vi "Audio Test.Generate Sine Sweep, Finite Steps.vi"(8 "error in":errorcluster, 10 "Cal Data":path, 11 "Sine Sweep Params":T1={"Duration"=2.1, "Amplitude"=1.0, "FreqStart"=20000.0, "FreqEnd"=100.0, "SampleRate"=44100.0, "StepCnt"=120, "FreqSpacing"=enum."Logarithmic", "Settling"={"Time"=0.0, "Cycles"=1.0}, "Measurement"={"Time"=0.001, "Cycles"=10.0}, "SyncPulseEn"=FALSE} {"Measurement"."Cycles" min=5.0 max=1000.0 step=1.0; "Measurement"."Time" min=0.0 max=5.0 step=0.0001 format="%.3f s"; "Settling"."Cycles" min=0.0 max=100.0 step=0.5; "Settling"."Time" min=0.0 max=5.0 step=0.0001 format="%.3f s"; "StepCnt" min=1; "Amplitude" min=0.0 max=1.0 step=0.1}) -> (0 "error out":errorcluster, 1 "Total Samples":i32, 2 "Output Wvfrm":waveform(dbl)(graph), 3 "SigConfig":refnum<class "SV Discrete Sweep.lvclass">, 4 "Cal Output Wvfrm":waveform(dbl)(graph))   [LabVIEW 2018]
uses:
  TypeDefs/AudioTest.Config, Sine Sweep Params_V2.ctl
  <vilib>/addons/_NISVFA/_Generation/Signal Generation/SV Discrete Sweep/SV Discrete Sweep.lvclass
  C:/Program Files (x86)/National Instruments/LabVIEW 2018/vi.lib/addons/_NISVFA/_Generation/Signal Generation/SV Signal/SV Signal.lvclass
  C:/Program Files (x86)/National Instruments/LabVIEW 2018/vi.lib/addons/_NISVFA/_Generation/Signal Generation/SV Function/SV Function.lvclass
  <vilib>/addons/_NISVFA/_Generation/Signal Generation/SV Signal/SV Signal.lvclass/SV Signal.ctl
  <vilib>/addons/_NISVFA/_Generation/Signal Generation/SV Discrete Sweep/SV Discrete Sweep.lvclass/SV Discrete Sweep.ctl
  <vilib>/addons/_NISVFA/_Generation/Signal Generation/SV Signal/Write Leading Synchronization Pulse Enable.vi
  <vilib>/addons/_NISVFA/_Generation/Signal Generation/SV Signal/Write Synchronization Pulse Duration.vi
  <vilib>/addons/_NISVFA/_Generation/Signal Generation/SV Signal/Write Synchronization Pulse Level.vi
  <vilib>/addons/_NISVFA/_Generation/Signal Generation/SV Signal/Write Synchronization Pulse Type.vi
  <vilib>/addons/_NISVFA/_Generation/Signal Generation/SV Discrete Sweep/Read All Frequencies and Amplitudes.vi
  <vilib>/addons/_NISVFA/_Generation/Signal Generation/SV Discrete Sweep/Write All Frequencies and Amplitudes.vi
  <vilib>/addons/_NISVFA/_Generation/Signal Generation/SV Discrete Sweep/Read Frequencies and Amplitudes.vi
  <vilib>/addons/_NISVFA/_Generation/Signal Generation/SV Discrete Sweep/Configure Frequency Sweep at Constant Amplitude.vi
  <vilib>/addons/_NISVFA/_Generation/Signal Generation/SV Signal/Write Ramp Parameters.vi
  <vilib>/addons/_NISVFA/_Generation/Signal Generation/SV Signal/Write DC Offset.vi
  <vilib>/addons/_NISVFA/_Generation/Signal Generation/SV Signal/Write Measurement Duration.vi
  <vilib>/addons/_NISVFA/_Generation/Signal Generation/SV Function/Write Measurement Cycles.vi
  <vilib>/addons/_NISVFA/_Generation/Signal Generation/SV Signal/Write Pre-Measurement Settling Duration.vi
  <vilib>/addons/_NISVFA/_Generation/Signal Generation/SV Function/Write Pre-Measurement Settling Cycles.vi
  <vilib>/addons/_NISVFA/_Generation/Signal Generation/SV Signal/Write Sample Rate.vi
  <vilib>/addons/_NISVFA/_Generation/Signal Generation/SV Signal/SV Signal.lvclass
panel:
  out "size(s)":i32
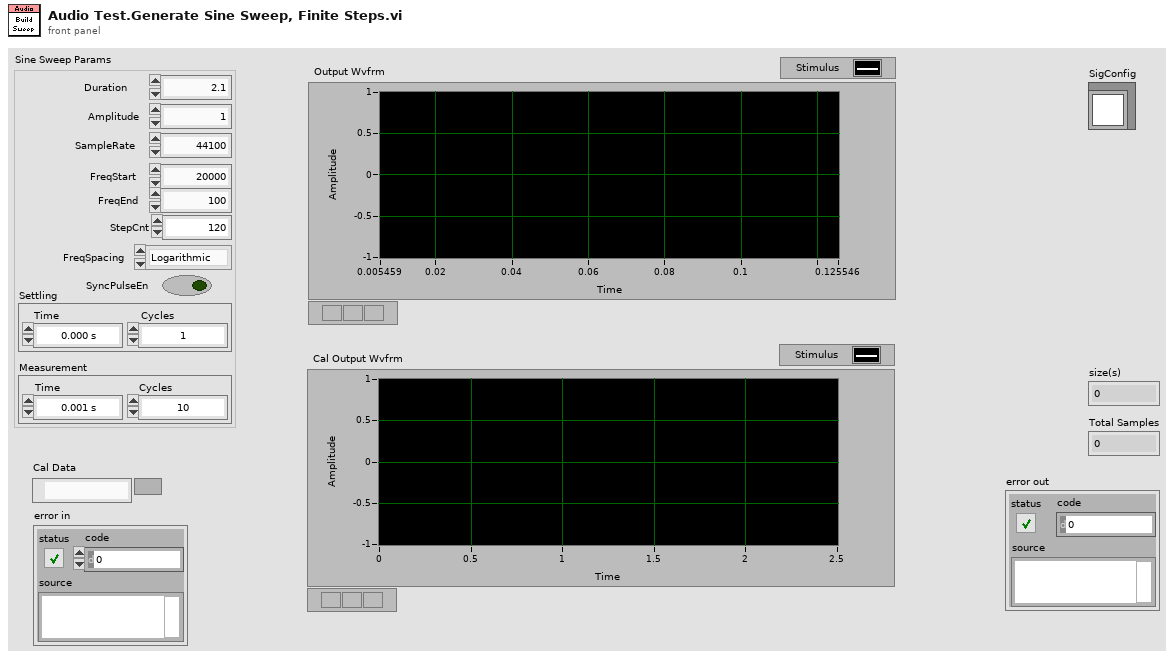
[diagram p1: front panel]
types:
  T1 = typedef "AudioTest.Config, Sine Sweep Params_V2.ctl" = cluster{"Duration":dbl, "Amplitude":dbl, "FreqStart":dbl, "FreqEnd":dbl, "SampleRate":dbl, "StepCnt":i32, "FreqSpacing":enum16{"Linear", "Logarithmic"}, "Settling":cluster{"Time":dbl, "Cycles":dbl}, "Measurement":cluster{"Time":dbl, "Cycles":dbl}, "SyncPulseEn":bool}
  T2 = enum16{"Noise", "MLS", "Chirp", "Monopulse", "Custom"}
  T3 = cluster{"profile":enum16{"Linear", "Half cosine"}, "durations [s]":cluster{"ramp-up":dbl, "transition":dbl, "ramp-down":dbl}}
  T4 = cluster{"frequency [Hz]":dbl, "amplitude [V]":dbl}[]
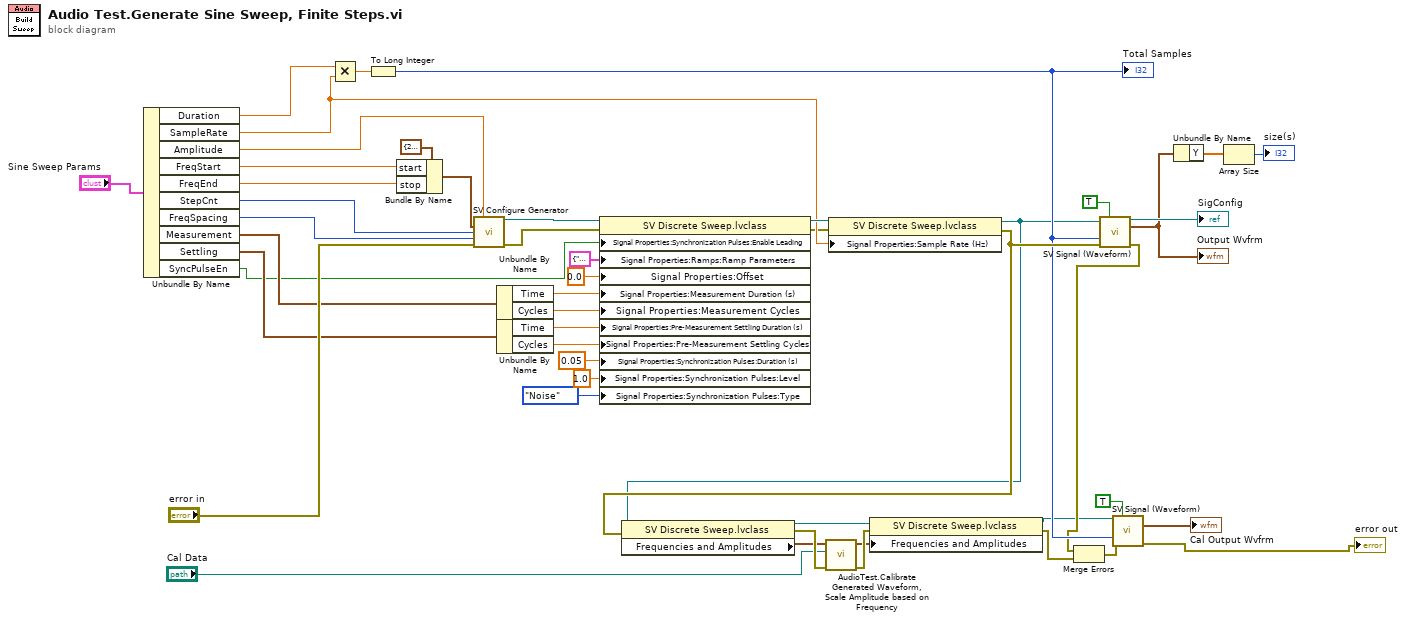
[diagram p0: block diagram]
diagram:
  n1 = Unbundle By Name("Sine Sweep Params") -> ("Duration"=w28:dbl, "SampleRate"=w29:dbl, "Amplitude"=w36:dbl, "FreqStart"=w38:dbl, "FreqEnd"=w37:dbl, "StepCnt"=w34:i32, "FreqSpacing"=w33:enum16{"Linear", "Logarithmic"}, "Measurement"=w32:cluster{"Time":dbl, "Cycles":dbl}, "Settling"=w31:cluster{"Time":dbl, "Cycles":dbl}, "SyncPulseEn"=w1:bool)
  n2 = Multiply(x=w28, y=w29) -> (x*y=w27:dbl)
  n3 = To Long Integer(number=w27) -> (32bit integer=w20:i32)
  "Total Samples" <- w20
  n4 = Bundle By Name(cluster=cluster{"start":dbl, "stop":dbl} {"start"=20000.0, "stop"=100.0} ("sweep range"), "start"=w38, "stop"=w37) -> (w39:cluster{"start":dbl, "stop":dbl})
  n5 = call-poly <vilib>:"SV Configure Generator.vi"("amplitude"=w36, "frequency range [Hz]"=w39, "number of steps"=w34, "profile"=w33, "error in (no error)"="error in") -> ("signal configuration"=w48:refnum<class "SV Discrete Sweep.lvclass">, "error out"=w42:errorcluster)  [unwired: 9 in]
  n6 = Unbundle By Name(w32) -> ("Time"=w44:dbl, "Cycles"=w43:dbl)
  n7 = Unbundle By Name(w31) -> ("Time"=w46:dbl, "Cycles"=w45:dbl)
  n8 = property class="SV Discrete Sweep.lvclass"(reference=w48, error in=w42, "Signal Properties:Synchronization Pulses:Enable Leading"=w1, "Signal Properties:Ramps:Ramp Parameters"=T3 {"profile"=enum."Half cosine", "durations [s]"={"ramp-up"=0.01, "transition"=0.0, "ramp-down"=0.01}} ("Ramp Parameters"), "Signal Properties:Offset"=0.0 ("DC offset [V]"), "Signal Properties:Measurement Duration (s)"=w44, "Signal Properties:Measurement Cycles"=w43, "Signal Properties:Pre-Measurement Settling Duration (s)"=w46, "Signal Properties:Pre-Measurement Settling Cycles"=w45, "Signal Properties:Synchronization Pulses:Duration (s)"=0.05 ("Synchronization Pulses:Duration"), "Signal Properties:Synchronization Pulses:Level"=1.0 ("Synchronization Pulses:Level"), "Signal Properties:Synchronization Pulses:Type"=T2."Noise" ("Synchronization Pulses:Type")) -> (reference out=w30:refnum<class "SV Discrete Sweep.lvclass">, error out=w25:errorcluster)
  n9 = property class="SV Discrete Sweep.lvclass"(reference=w30, error in=w25, "Signal Properties:Sample Rate (Hz)"=w29) -> (reference out=w13:refnum<class "SV Discrete Sweep.lvclass">, error out=w24:errorcluster)
  n10 = property class="SV Discrete Sweep.lvclass"(reference=w13, error in=w24) -> (reference out=w23:refnum<class "SV Discrete Sweep.lvclass">, error out=w22:errorcluster, "Frequencies and Amplitudes"=w14:T4)
  n11 = call "AudioTest.Calibrate Generated Waveform, Scale Amplitude based on Frequency.vi"("error in (no error)"=w22, "Calibration File"="Cal Data", "Frequencies and Amplitudes"=w14) -> ("error out"=w21:errorcluster, "Frequencies and Amplitudes Out"=w12:T4)  [unwired: 7 in]
  n12 = property class="SV Discrete Sweep.lvclass"(reference=w23, error in=w21, "Frequencies and Amplitudes"=w12) -> (reference out=w11:refnum<class "SV Discrete Sweep.lvclass">, error out=w16:errorcluster)
  n13 = call-dynamic "SV Signal (Waveform).vi"("signal configuration"=w13, "reset"=TRUE, "samples"=w20, "error in (no error)"=w24) -> ("signal configuration"=→"SigConfig":refnum<class "SV Discrete Sweep.lvclass">, "output waveform"=w10:waveform(dbl), "error out"=w17:errorcluster)  [unwired: 6 in, 3 out]
  "Output Wvfrm" <- w10
  n14 = Merge Errors(w17, w16) -> (w6:errorcluster)
  n15 = call-dynamic "SV Signal (Waveform).vi"("signal configuration"=w11, "reset"=TRUE, "samples"=w20, "error in (no error)"=w6) -> ("output waveform"=→"Cal Output Wvfrm":waveform(dbl), "error out"=→"error out":errorcluster)  [unwired: 6 in, 4 out]
  n16 = Unbundle By Name(w10) -> ("Y"=w9:dbl[])
  n17 = Array Size(array=w9) -> (size(s)=→"size(s)":i32)
